vi "SubDrawTextPix2World.vi"(0 "Calibration Template Image Out":T1, 1 "X Y Pixel Co-Ordinate":cluster{sgl, sgl}, 3 "Refnum Img Out":T1) -> (6 "X Y World Co-Ordinate":cluster{sgl, sgl})   [LabVIEW 2015]
uses:
  <vilib>/vision/Image Controls.llb/IMAQ Image.ctl
  <vilib>/vision/NI_Vision_Development_Module.lvlib
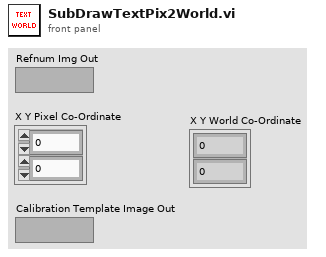
[diagram p1: front panel]
types:
  T1 = typedef "IMAQ Image.ctl" = refnum<image>
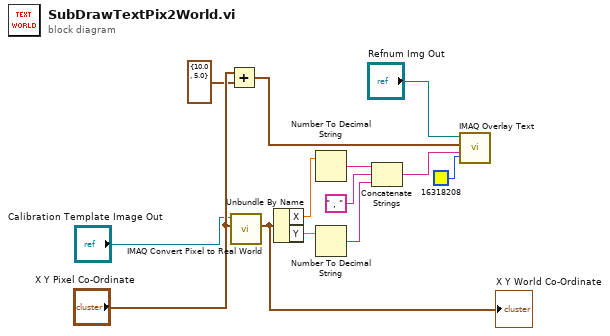
[diagram p0: block diagram]
diagram:
  n1 = Add(x="X Y Pixel Co-Ordinate", y=cluster{"x":sgl, "y":sgl} {"x"=10.0, "y"=5.0}) -> (x+y=w8:cluster{sgl, sgl})
  n2 = call "IMAQ Convert Pixel to Real World"("Pixel Coordinates"="X Y Pixel Co-Ordinate", "Calibrated Image"="Calibration Template Image Out") -> ("Real World Coordinates"=w1:cluster{"X":sgl, "Y":sgl})  [unwired: 4 in, 5 out]
  "X Y World Co-Ordinate" <- w1
  n3 = Unbundle By Name(w1) -> ("X"=w10:sgl, "Y"=w11:sgl)
  n4 = Number To Decimal String(number=w10) -> (decimal integer string=w3:string)  [unwired: 1 in]
  n5 = Number To Decimal String(number=w11) -> (decimal integer string=w4:string)  [unwired: 1 in]
  n6 = Concatenate Strings(w3, " , " ("string"), w4) -> (w6:string)
  n7 = call "IMAQ Overlay Text"("Text Color (black)"=u32 16318208, "String"=w6, "Origin"=w8, "Image"="Refnum Img Out") -> ()  [unwired: 6 in, 2 out]
